vi "ex_getDAQmxAttrFromRcFile.vi"(8 "error in (no error)":errorcluster) -> (0 "error out":errorcluster, 3 "Classes":T1[](array[typedef])=[{"Name"="", "Local Name"="", "Generic Type"="", "Super"=[], "Forward Declare Class"=FALSE, "Flags"=0, "Generic Type Property Overrides"={"Refnum Kind"=enum."noRefNum", "Set Function"="", "Get Function"="", "Library Name"="", "Control Name"="", "Diagram Control Resource ID"=0, "Panel Control Resource ID"=0, "Open Function"="", "Close Function"="", "Cleanup Proc"=enum."noCleanup", "Open Function Takes Context"=enum."default", "Session Library Name"="", "Reset Function"="", "Duplicate Function"="", "Flatten Function"="", "Unflatten Function"="", "Mutate From Control"="", "Class Info Function"="", "Source Palette Item"="", "Terminal Name"="", "Event Register Function"="", "Event Unregister Function"="", "Event Error Passing"=enum."noErrorPassing", "Has Active Property"=enum."no", "Attribute Error Passing"=enum."noErrorPassing", "Method Error Passing"=enum."noErrorPassing", "Adapt to Type"=enum."default", "Match Exact Type Descriptor"=enum."noMatching", "Show Select Menu Item"=enum."default", "Sorted Properties"=enum."default", "Calling Convention"=enum."noCalling", "Filtering"={"Type of Filtering"=enum."no filtering", "Filtering Dialog VI"="", "Popup Menu String"="", "Callback Function"=""}, "Non Zero Return Values As Errors"=enum."default"}, "Attributes"=[], "Methods"=[], "Events"=[], "Class Version"=0}, {"Name"="", "Local Name"="", "Generic Type"="", "Super"=[], "Forward Declare Class"=FALSE, "Flags"=0, "Generic Type Property Overrides"={"Refnum Kind"=enum."noRefNum", "Set Function"="", "Get Function"="", "Library Name"="", "Control Name"="", "Diagram Control Resource ID"=0, "Panel Control Resource ID"=0, "Open Function"="", "Close Function"="", "Cleanup Proc"=enum."noCleanup", "Open Function Takes Context"=enum."default", "Session Library Name"="", "Reset Function"="", "Duplicate Function"="", "Flatten Function"="", "Unflatten Function"="", "Mutate From Control"="", "Class Info Function"="", "Source Palette Item"="", "Terminal Name"="", "Event Register Function"="", "Event Unregister Function"="", "Event Error Passing"=enum."noErrorPassing", "Has Active Property"=enum."no", "Attribute Error Passing"=enum."noErrorPassing", "Method Error Passing"=enum."noErrorPassing", "Adapt to Type"=enum."default", "Match Exact Type Descriptor"=enum."noMatching", "Show Select Menu Item"=enum."default", "Sorted Properties"=enum."default", "Calling Convention"=enum."noCalling", "Filtering"={"Type of Filtering"=enum."no filtering", "Filtering Dialog VI"="", "Popup Menu String"="", "Callback Function"=""}, "Non Zero Return Values As Errors"=enum."default"}, "Attributes"=[], "Methods"=[], "Events"=[], "Class Version"=0}] {"Events"."Event Code" max=1073741823 step=1 format="%x"; "Methods"."Method Code" format="%x"; "Attributes"."Number of Dimensions" format="%x"; "Attributes"."Property Code" format="%x"})   [LabVIEW 2017]
uses:
  utility/RCeditor/rc editor utility.llb/rc editor utility.lvlib
  utility/RCeditor/rc editor read.llb/rc editor read.lvlib
  utility/RCeditor/rc editor controls.llb/typesettings.ctl
  utility/RCeditor/rc editor controls.llb/rc editor controls.lvlib
  utility/RCeditor/rc editor controls.llb/typeflags.ctl
  utility/RCeditor/rc editor controls.llb/enumeration.ctl
  utility/RCeditor/rc editor controls.llb/accessenum.ctl
  utility/RCeditor/rc editor controls.llb/datatypeenum.ctl
  utility/RCeditor/rc editor controls.llb/clustercontrol.ctl
  utility/RCeditor/rc editor controls.llb/yesnoenum.ctl
  utility/RCeditor/rc editor controls.llb/initnameformat.ctl
  utility/RCeditor/rc editor controls.llb/attribute3.ctl
  utility/RCeditor/rc editor controls.llb/numericdatatypeenum.ctl
  utility/RCeditor/rc editor controls.llb/stringdatatypeenum.ctl
  utility/RCeditor/rc editor controls.llb/passbyenum.ctl
  utility/RCeditor/rc editor controls.llb/arrayfmtenum.ctl
  utility/RCeditor/rc editor controls.llb/datanameenum.ctl
  utility/RCeditor/rc editor controls.llb/paraminoutenum.ctl
  utility/RCeditor/rc editor controls.llb/parameter2.ctl
  utility/RCeditor/rc editor controls.llb/methflagsenum.ctl
  utility/RCeditor/rc editor controls.llb/method3.ctl
  utility/RCeditor/rc editor controls.llb/yesnodefaultenum.ctl
  utility/RCeditor/rc editor controls.llb/cleanupenum.ctl
  utility/RCeditor/rc editor controls.llb/callingenum.ctl
  utility/RCeditor/rc editor controls.llb/errorpassingenum.ctl
  utility/RCeditor/rc editor controls.llb/dialogenum.ctl
  utility/RCeditor/rc editor controls.llb/filtering.ctl
  utility/RCeditor/rc editor controls.llb/matchexactenum.ctl
  utility/RCeditor/rc editor controls.llb/generictype3.ctl
  utility/RCeditor/rc editor controls.llb/eventparamtype.ctl
  utility/RCeditor/rc editor controls.llb/eventparam.ctl
  utility/RCeditor/rc editor controls.llb/eventdef.ctl
  utility/RCeditor/rc editor controls.llb/class3.ctl
  utility/RCeditor/rc editor controls.llb/refnumenum4.ctl
panel:
  in  "Type Settings":T30 {"Type Flags" items=["none", "verifyLibrary"]}
  out "Progress":dbl(slide) caption="Reading File" min=0.0 max=1.0 step=0.01 scale=0.0..1.0
  out "Class Names":string[](array[string])
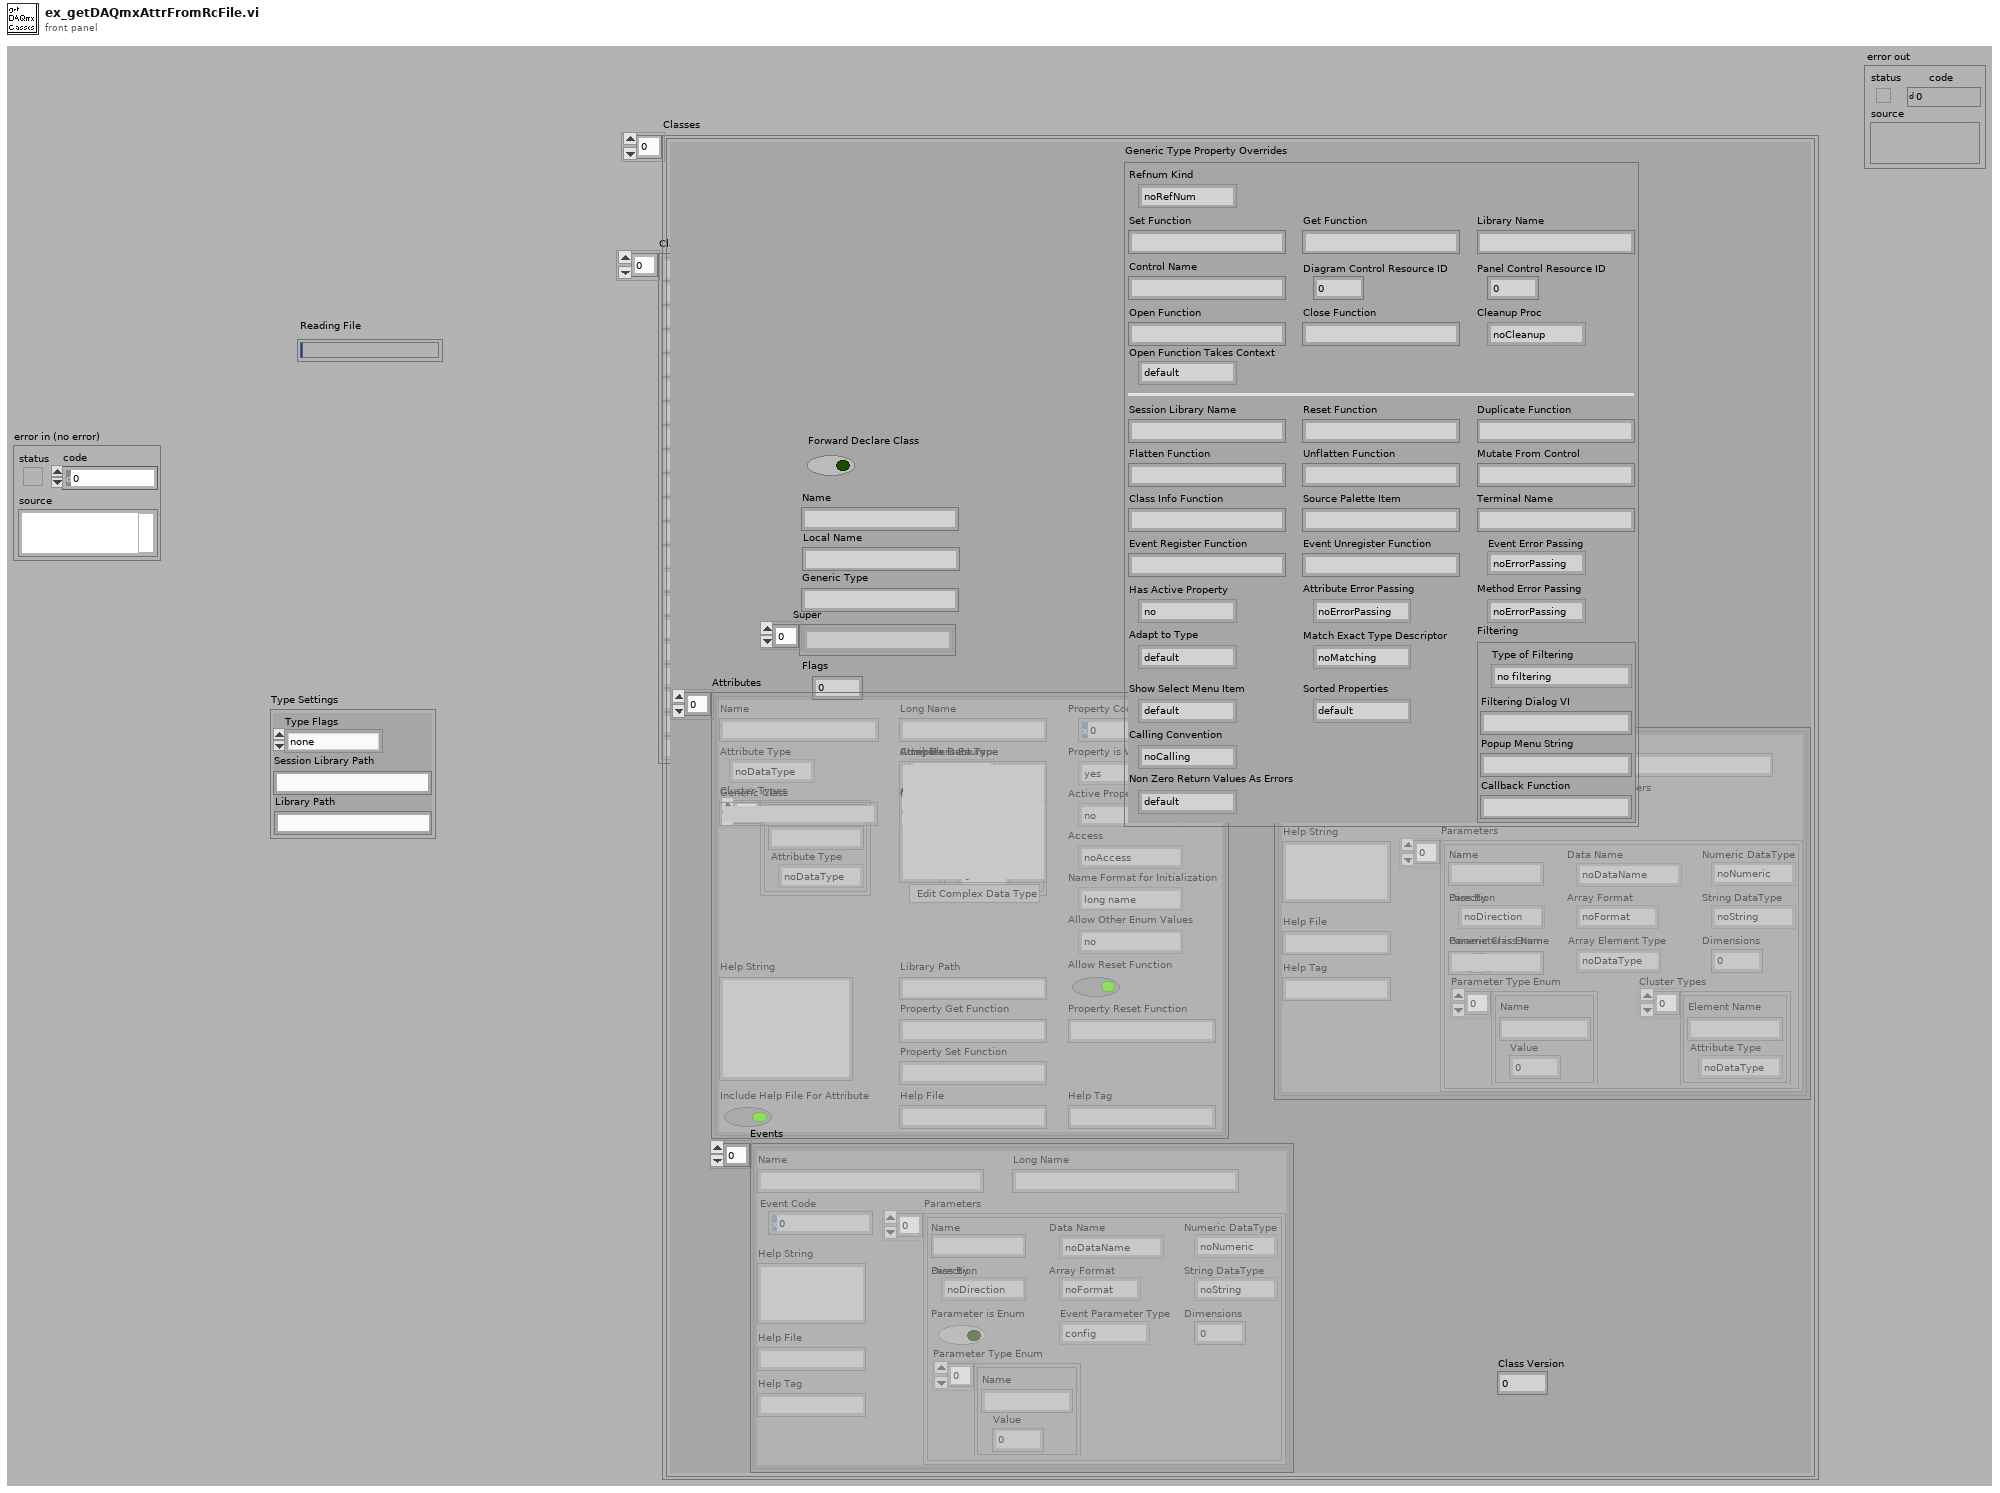
[diagram p1: front panel]
types:
  T1 = typedef "rc editor controls.lvlib/class3.ctl" = cluster{"Name":string, "Local Name":string, "Generic Type":string, "Super":string[], "Forward Declare Class":bool, "Flags":i32, "Generic Type Property Overrides":T2, "Attributes":T11[], "Methods":T18[], "Events":T27[], "Class Version":u32}
  T2 = typedef "rc editor controls.lvlib/generictype3.ctl" = cluster{"Refnum Kind":T3, "Set Function":string, "Get Function":string, "Library Name":string, "Control Name":string, "Diagram Control Resource ID":i32, "Panel Control Resource ID":i32, "Open Function":string, "Close Function":string, "Cleanup Proc":T4, "Open Function Takes Context":T5, "Session Library Name":string, "Reset Function":string, "Duplicate Function":string, "Flatten Function":string, "Unflatten Function":string, "Mutate From Control":string, "Class Info Function":string, "Source Palette Item":string, "Terminal Name":string, "Event Register Function":string, "Event Unregister Function":string, "Event Error Passing":T6, "Has Active Property":T5, "Attribute Error Passing":T6, "Method Error Passing":T6, "Adapt to Type":T5, "Match Exact Type Descriptor":T7, "Show Select Menu Item":T5, "Sorted Properties":T5, "Calling Convention":T8, "Filtering":T9, "Non Zero Return Values As Errors":T5}
  T3 = typedef "rc editor controls.lvlib/refnumenum4.ctl" = enum16{"noRefNum", "Refnum", "RefnumTag", "Tag", "RefnumTagByRefFlatten"}
  T4 = typedef "rc editor controls.lvlib/cleanupenum.ctl" = enum16{"noCleanup", "exit", "idle", "reset", "idleNotTop", "resetNotTop", "doNotCleanup"}
  T5 = typedef "rc editor controls.lvlib/yesnodefaultenum.ctl" = enum16{"default", "no", "yes"}
  T6 = typedef "rc editor controls.lvlib/errorpassingenum.ctl" = enum16{"noErrorPassing", "none", "stringFirst", "stringLast"}
  T7 = typedef "rc editor controls.lvlib/matchexactenum.ctl" = enum16{"noMatching", "none", "withInheritance", "strict"}
  T8 = typedef "rc editor controls.lvlib/callingenum.ctl" = enum16{"noCalling", "std", "C"}
  T9 = typedef "rc editor controls.lvlib/filtering.ctl" = cluster{"Type of Filtering":T10, "Filtering Dialog VI":string, "Popup Menu String":string, "Callback Function":string}
  T10 = typedef "rc editor controls.lvlib/dialogenum.ctl" = enum16{"no filtering", "filtering", "ipfiltering"}
  T11 = typedef "rc editor controls.lvlib/attribute3.ctl" = cluster{"Name":string, "Long Name":string, "Property Code":i32, "Attribute Type":T12, "Cluster Types":T13[], "Attribute is Enum":bool, "Attribute Type Enum":T14[], "Property is Visible":T15, "Active Property":T15, "Access":T16, "Help String":string, "Library Path":string, "Property Get Function":string, "Property Set Function":string, "Allow Reset Function":bool, "Property Reset Function":string, "Generic Class":string, "Allow Other Enum Values":T15, "Array Element Type":T12, "Number of Dimensions":i32, "Complex Data Type":string, "Edit Complex Data Type":bool, "Name Format for Initialization":T17, "Include Help File For Attribute":bool, "Help Tag":string, "Help File":string}
  T12 = typedef "rc editor controls.lvlib/datatypeenum.ctl" = enum16{"noDataType", "void", "iB", "iW", "iL", "iQ", "uB", "uW", "uL", "uQ", "fS", "fS1D", "fD", "fD1D", "bool", "bool1D", "string", "string1D", "path", "rect", "point", "VIRef", "VIRefReservation", "file", "VIExecState", "htmlImgFmt", "printFmt", "iW1D", "uW1D", "iL1D", "uL1D", "iQ1D", "uQ1D", "uB1D", "iB1D", "VisaRef", "DAQChannel", "DAQDevice", "DAQPhysChan", "DAQScale", "DAQSwitch", "DAQTask", "DAQTerminal", "DAQTrigger", "cluster", "genclass", "timestamp", "array", "variant", "complex type"}
  T13 = typedef "rc editor controls.lvlib/clustercontrol.ctl" = cluster{"Element Name":string, "Attribute Type":T12}
  T14 = typedef "rc editor controls.lvlib/enumeration.ctl" = cluster{"Name":string, "Value":i32}
  T15 = typedef "rc editor controls.lvlib/yesnoenum.ctl" = enum16{"no", "yes"}
  T16 = typedef "rc editor controls.lvlib/accessenum.ctl" = enum16{"noAccess", "readwrite", "readonly", "writeonly"}
  T17 = typedef "rc editor controls.lvlib/initnameformat.ctl" = enum16{"long name", "short name"}
  T18 = typedef "rc editor controls.lvlib/method3.ctl" = cluster{"Name":string, "Local Name":string, "Method Flags":T19, "Method Code":i32, "# Optional Parameters":i32, "Parameters":T20[], "Help String":string, "Help Tag":string, "Help File":string}
  T19 = typedef "rc editor controls.lvlib/methflagsenum.ctl" = enum16{"noFlags", "noInvoke", "returnValue", "returnErrClustCode", "0", "retErrClustNoInv"}
  T20 = typedef "rc editor controls.lvlib/parameter2.ctl" = cluster{"Name":string, "Data Name":T21, "Numeric DataType":T22, "String DataType":T23, "Dimensions":u32, "Pass By":T24, "Array Format":T25, "Parameter is Enum":bool, "Parameter Type Enum":T14[], "Cluster Types":T13[], "Generic Class Name":string, "Array Element Type":T12, "Direction":T26}
  T21 = typedef "rc editor controls.lvlib/datanameenum.ctl" = enum16{"noDataName", "numeric", "array", "string", "void", "error", "cluster", "genclass", "timestamp", "variant", "non numeric array", "bool", "path"}
  T22 = typedef "rc editor controls.lvlib/numericdatatypeenum.ctl" = enum16{"noNumeric", "int8", "int16", "int32", "int64", "uInt8", "uInt16", "uInt32", "uInt64", "single", "double"}
  T23 = typedef "rc editor controls.lvlib/stringdatatypeenum.ctl" = enum16{"noString", "CStr", "PStr", "StrHandle", "StrHandlePtr"}
  T24 = typedef "rc editor controls.lvlib/passbyenum.ctl" = enum16{"noPassing", "value", "reference", "refInOut"}
  T25 = typedef "rc editor controls.lvlib/arrayfmtenum.ctl" = enum16{"noFormat", "pointer", "handle", "handlepointer"}
  T26 = typedef "rc editor controls.lvlib/paraminoutenum.ctl" = enum16{"noDirection", "in", "out", "inout"}
  T27 = typedef "rc editor controls.lvlib/eventdef.ctl" = cluster{"Name":string, "Long Name":string, "Event Code":u32, "Parameters":T28[], "Help String":string, "Help Tag":string, "Help File":string}
  T28 = typedef "rc editor controls.lvlib/eventparam.ctl" = cluster{"Name":string, "Data Name":T21, "Numeric DataType":T22, "String DataType":T23, "Dimensions":u32, "Pass By":T24, "Array Format":T25, "Parameter is Enum":bool, "Parameter Type Enum":T14[], "Direction":T26, "Event Parameter Type":T29}
  T29 = typedef "rc editor controls.lvlib/eventparamtype.ctl" = enum16{"config", "data", "configdata"}
  T30 = typedef "rc editor controls.lvlib/typesettings.ctl" = cluster{"Type Flags":T31, "Session Library Path":string, "Library Path":string}
  T31 = typedef "rc editor controls.lvlib/typeflags.ctl" = u32
  T32 = typedef "class3.ctl" = cluster{"Name":string, "Local Name":string, "Generic Type":string, "Super":string[], "Forward Declare Class":bool, "Flags":i32, "Generic Type Property Overrides":T33, "Attributes":T42[], "Methods":T49[], "Events":T58[]}
  T33 = typedef "generictype3.ctl" = cluster{"Refnum Kind":T34, "Set Function":string, "Get Function":string, "Library Name":string, "Control Name":string, "Diagram Control Resource ID":i32, "Panel Control Resource ID":i32, "Open Function":string, "Close Function":string, "Cleanup Proc":T35, "Open Function Takes Context":T36, "Session Library Name":string, "Reset Function":string, "Duplicate Function":string, "Flatten Function":string, "Unflatten Function":string, "Mutate From Control":string, "Class Info Function":string, "Source Palette Item":string, "Terminal Name":string, "Event Register Function":string, "Event Unregister Function":string, "Event Error Passing":T37, "Has Active Property":T36, "Attribute Error Passing":T37, "Method Error Passing":T37, "Adapt to Type":T36, "Match Exact Type Descriptor":T38, "Show Select Menu Item":T36, "Sorted Properties":T36, "Calling Convention":T39, "Filtering":T40, "Non Zero Return Values As Errors":T36}
  T34 = typedef "refnumenum.ctl" = enum16{"noRefNum", "Generic", "GenericTag", "GenericByValue", "GenericByRefFlatten", "GenericTagByRefFlatten"}
  T35 = typedef "cleanupenum.ctl" = enum16{"noCleanup", "exit", "idle", "reset", "idleNotTop", "resetNotTop", "doNotCleanup"}
  T36 = typedef "yesnodefaultenum.ctl" = enum16{"default", "no", "yes"}
  T37 = typedef "errorpassingenum.ctl" = enum16{"noErrorPassing", "none", "stringFirst", "stringLast"}
  T38 = typedef "matchexactenum.ctl" = enum16{"noMatching", "none", "withInheritance", "strict"}
  T39 = typedef "callingenum.ctl" = enum16{"noCalling", "std", "C"}
  T40 = typedef "filtering.ctl" = cluster{"Type of Filtering":T41, "Filtering Dialog VI":string, "Popup Menu String":string, "Callback Function":string}
  T41 = typedef "dialogenum.ctl" = enum16{"no filtering", "filtering", "ipfiltering"}
  T42 = typedef "attribute3.ctl" = cluster{"Name":string, "Long Name":string, "Property Code":i32, "Attribute Type":T43, "Cluster Types":T44[], "Attribute is Enum":bool, "Attribute Type Enum":T45[], "Property is Visible":T46, "Active Property":T46, "Access":T47, "Help String":string, "Library Path":string, "Property Get Function":string, "Property Set Function":string, "Allow Reset Function":bool, "Property Reset Function":string, "Generic Class":string, "Allow Other Enum Values":T46, "Array Element Type":T43, "Number of Dimensions":i32, "Complex Data Type":string, "Edit Complex Data Type":bool, "Name Format for Initialization":T48, "Include Help File For Attribute":bool, "Help Tag":string, "Help File":string}
  T43 = typedef "datatypeenum.ctl" = enum16{"noDataType", "void", "iB", "iW", "iL", "iQ", "uB", "uW", "uL", "uQ", "fS", "fS1D", "fD", "fD1D", "bool", "bool1D", "string", "string1D", "path", "rect", "point", "VIRef", "VIRefReservation", "file", "VIExecState", "htmlImgFmt", "printFmt", "iW1D", "uW1D", "iL1D", "uL1D", "iQ1D", "uQ1D", "uB1D", "iB1D", "VisaRef", "DAQChannel", "DAQDevice", "DAQPhysChan", "DAQScale", "DAQSwitch", "DAQTask", "DAQTerminal", "DAQTrigger", "cluster", "genclass", "timestamp", "array", "variant", "complex type"}
  T44 = typedef "clustercontrol.ctl" = cluster{"Element Name":string, "Attribute Type":T43}
  T45 = typedef "enumeration.ctl" = cluster{"Name":string, "Value":i32}
  T46 = typedef "yesnoenum.ctl" = enum16{"no", "yes"}
  T47 = typedef "accessenum.ctl" = enum16{"noAccess", "readwrite", "readonly", "writeonly"}
  T48 = typedef "initnameformat.ctl" = enum16{"long name", "short name"}
  T49 = typedef "method3.ctl" = cluster{"Name":string, "Local Name":string, "Method Flags":T50, "Method Code":i32, "# Optional Parameters":i32, "Parameters":T51[], "Help String":string, "Help Tag":string, "Help File":string}
  T50 = typedef "methflagsenum.ctl" = enum16{"noFlags", "noInvoke", "returnValue", "returnErrClustCode", "0", "retErrClustNoInv"}
  T51 = typedef "parameter2.ctl" = cluster{"Name":string, "Data Name":T52, "Numeric DataType":T53, "String DataType":T54, "Dimensions":u32, "Pass By":T55, "Array Format":T56, "Parameter is Enum":bool, "Parameter Type Enum":T45[], "Cluster Types":T44[], "Generic Class Name":string, "Array Element Type":T43, "Direction":T57}
  T52 = typedef "datanameenum.ctl" = enum16{"noDataName", "numeric", "array", "string", "void", "error", "cluster", "genclass", "timestamp", "variant", "non numeric array", "bool", "path"}
  T53 = typedef "numericdatatypeenum.ctl" = enum16{"noNumeric", "int8", "int16", "int32", "int64", "uInt8", "uInt16", "uInt32", "uInt64", "single", "double"}
  T54 = typedef "stringdatatypeenum.ctl" = enum16{"noString", "CStr", "PStr", "StrHandle", "StrHandlePtr"}
  T55 = typedef "passbyenum.ctl" = enum16{"noPassing", "value", "reference", "refInOut"}
  T56 = typedef "arrayfmtenum.ctl" = enum16{"noFormat", "pointer", "handle", "handlepointer"}
  T57 = typedef "paraminoutenum.ctl" = enum16{"noDirection", "in", "out", "inout"}
  T58 = typedef "eventdef.ctl" = cluster{"Name":string, "Long Name":string, "Event Code":u32, "Parameters":T59[], "Help String":string, "Help Tag":string, "Help File":string}
  T59 = typedef "eventparam.ctl" = cluster{"Name":string, "Data Name":T52, "Numeric DataType":T53, "String DataType":T54, "Dimensions":u32, "Pass By":T55, "Array Format":T56, "Parameter is Enum":bool, "Parameter Type Enum":T45[], "Direction":T57, "Event Parameter Type":T60}
  T60 = typedef "eventparamtype.ctl" = enum16{"config", "data", "configdata"}
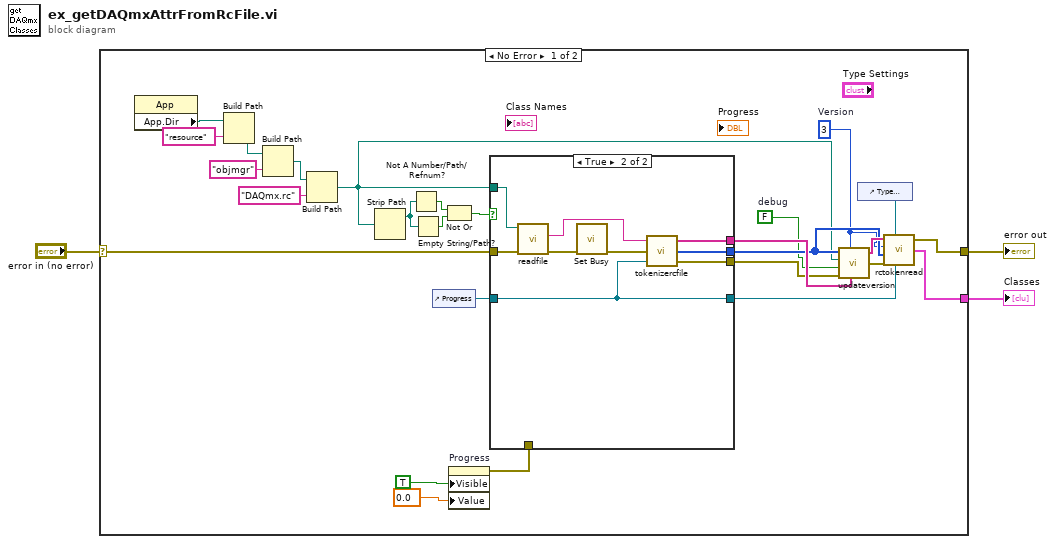
[diagram p0: block diagram]
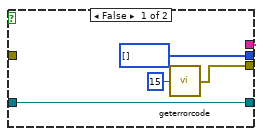
[diagram p2: hidden frame]
diagram:
  n1 = case shown="No Error" "error in (no error)" {
    selector: "error in (no error)" -> [w11 w45]
    tunnel: [w13 _] -> w3
    tunnel: [w12 w45] -> w2
    frame No Error {
      w14 = FALSE  # debug
      w15 = 3  # Version
      n2 = property class="App"() -> ("App.Dir"=w10:path)  [unwired: 2 in, 2 out]
      n3 = Build Path(base path=w10, name or relative path="resource") -> (appended path=w7:path)
      n4 = Build Path(base path=w7, name or relative path="objmgr") -> (appended path=w5:path)
      n5 = Build Path(base path=w5, name or relative path="DAQmx.rc") -> (appended path=w4:path)
      n6 = Strip Path(path=w4) -> (stripped path=w30:path)  [unwired: 1 out]
      n7 = Not A Number/Path/Refnum?(number/path/refnum=w30) -> (NaN/Path/Refnum?=w29:bool)
      n8 = Empty String/Path?(string/path=w30) -> (empty?=w28:bool)
      n9 = control-ref of="Progress"() -> (w19:refnum<vi>)
      n10 = Not Or(1:w28, 2:w29) -> (0:w27:bool)
      n11 = property on="Progress" class="Slide (strict)"("Visible"=TRUE, "Value"=0.0 ("Progress")) -> (error out=w20:errorcluster)  [unwired: 2 in, 1 out]
      n12 = case shown="True" w27 {
        tunnel: [string[] [] ("String Array") w44] -> w26
        tunnel: [w31 w43] -> w18
        tunnel: w4 -> [_ w42]
        tunnel: [i32[] [] ("Line Number Array") w40] -> w23
        tunnel: w20 -> [_ _]
        tunnel: w19 -> [w33 w39]
        tunnel: [w33 w39] -> w17
        tunnel: w11 -> [_ w36]
        frame False {
          n13 = call "geterrorcode.vi"("index"=15 ("code")) -> ("Error String"=w31:errorcluster)
        }
        frame True {
          n14 = call "readfile.vi"("error in (no error)"=w36, "file path (dialog if empty)"=w42) -> ("error out"=w37:errorcluster, "character string"=w41:string)  [unwired: 5 in, 3 out]
          n15 = call <vilib>:"Set Busy.vi"("error in (no error)"=w37) -> ("error out"=w38:errorcluster)  [unwired: 9 in, 1 out]
          n16 = call "tokenizercfile.vi"("Slide Refnum"=w39, "error in"=w38, "String"=w41) -> ("error out"=w43:errorcluster, "Line Number Array"=w40:i32[], "String Array"=w44:string[])
        }
      }
      n17 = call "updateversion.vi"("Line Number Array"=w23, "Version"=w15, "Path"=w4, "debug"=w14, "String Array"=w26, "error out"=w18) -> ("String Array 2"=w24:string[], "error IO"=w25:errorcluster)  [unwired: 1 out]
      n18 = control-ref of="Type Settings"() -> (w16:refnum<vi>)
      n19 = call "rctokenread.vi"("String Array"=w24, "Type Settings  Refnum"=w16, "Version"=w15, "Line Number Array"=w23, "Progress"=w17, "error IO"=w25) -> ("error"=w12:errorcluster, "Classes"=w13:T32[])  [unwired: 1 out]
    }
    frame Error {
    }
  }
  "error out" <- w2
  "Classes" <- w3
